vi "SVT Get Octave Value.vi"   [LabVIEW 2017, in "SoundVib_Octave_2014 standard.lvlib"]
doc: "Extracts the band power value of the <B>octave spectrum</B> at the specified input frequency. Finds the octave band that corresponds to the input frequency if the input frequency does not exactly coincide with a nominal frequency. Wire data to the <B>octave spectrum</B> input to determine the polymorphic instance to use or manually select the instance."
uses:
  <vilib>/addons/Sound and Vibration/svt_Octave/SoundVib_Octave_2014 standard.lvlib
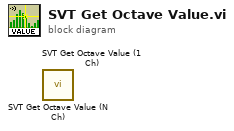
[diagram p0: block diagram]
diagram:
  n1 = call <vilib>:"SVT Get Octave Value (N Ch).vi"() -> ()  [unwired: 12 in, 4 out]
  n2 = call <vilib>:"SVT Get Octave Value (1 Ch).vi"() -> ()  [unwired: 12 in, 4 out]
